vi "SpaceVectorCalc.vi"(0 "ref_alpha":sgl caption="voltage alpha", 1 "Resources":T1={"Multiplier"=refnum, "Divider"=refnum, "Adder"=refnum}, 2 "Parameters":T2={"Deadtime"="Deadtime", "Period"="Period", "A_timing"="A_timing", "B_timing"="B_timing", "C_timing"="C_timing"}, 5 "ref_beta":sgl caption="voltage beta", 7 "ref_max":sgl=1.0) -> (4 "SVPWM_Timing":cluster{"ON":u32, "OFF":u32}[](array[cluster]), 15 "SVPWM_Sector":u8)   [LabVIEW 2017, in "SVPWM.lvlib"]
uses:
  SVPWM.lvlib
  Parameters.ctl
  <vilib>/NI/NonreentrantSinglePoint/Multiplier/Multiplier.lvclass
  <vilib>/NI/NonreentrantSinglePoint/Divider/Divider.lvclass
  <vilib>/NI/NonreentrantSinglePoint/Adder/Adder.lvclass
  <vilib>/rvi/DataTransferAndStorage/Container/Common/niFpgaContainerExecOnDevCompGetState.vi
  <vilib>/rvi/Emulation/niFpgaEmulationIsFPGAContextNoSignature.vi
  <vilib>/rvi/DataTransferAndStorage/Container/Common/niFpgaContainerGetUniqueNameForEmu.vi
  <vilib>/rvi/Memory/Memory_Emulation/niFpgaMemoryEmulationCacheClearOnFirstRun.vi
  <vilib>/rvi/Memory/Memory_Emulation/nirvimemoryEmulationManagerCache_MakeExclusive.vi
  <vilib>/rvi/Memory/Memory_Emulation/niFpgaMemoryEmulationValidateCache.vi
  <vilib>/rvi/Memory/Memory_Emulation/nirvimemoryEmulationManagerCache_InsertValue.vi
  <vilib>/Utility/error.llb/Clear Errors.vi
  <vilib>/rvi/Memory/Memory_Emulation/nirvimemoryEmulationManagerCache_ReleaseExclusive.vi
  <vilib>/rvi/Memory/Memory_Emulation/nirvimemoryEmulationManagerCache_GetValue.vi
  <vilib>/rvi/Memory/Memory_Emulation/nirvimemoryEmulationManagerCache_SetValue.vi
  <vilib>/rvi/Emulation/niFpgaProcessEmulError.vi
  <vilib>/rvi/Emulation/niFpgaSctlEmulationGetInTimedLoop.vi
  <vilib>/rvi/DataTransferAndStorage/Container/XNode/niFpgaContainer.xnode
  <vilib>/rvi/DataTransferAndStorage/Register/Emulation/niFpgaRegisterEmulationRefIn.vi
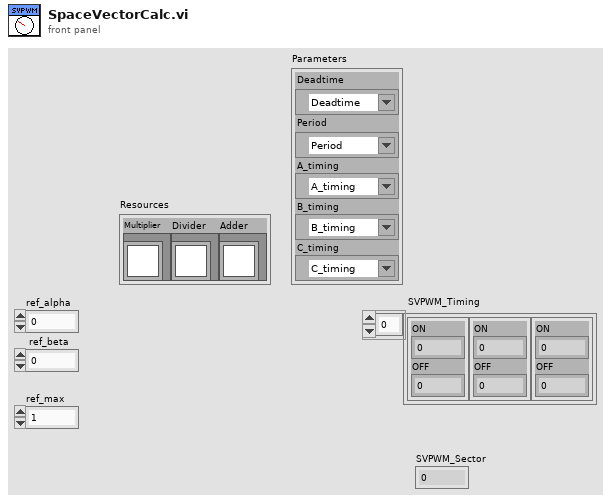
[diagram p1: front panel]
types:
  T1 = cluster{"Multiplier":refnum<class "Multiplier.lvclass">, "Divider":refnum<class "Divider.lvclass">, "Adder":refnum<class "Adder.lvclass">}
  T2 = typedef "SVPWM.lvlib/Parameters.ctl" = cluster{"Deadtime":refnum<k21>, "Period":refnum<k21>, "A_timing":refnum<k21>, "B_timing":refnum<k21>, "C_timing":refnum<k21>}
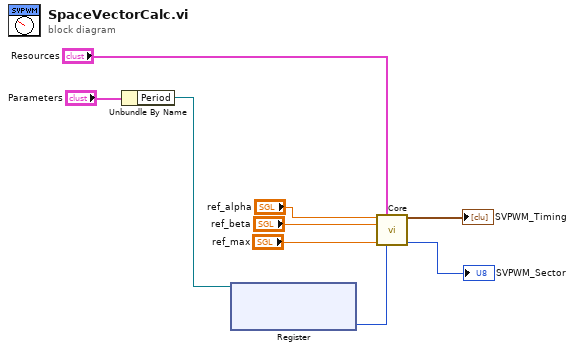
[diagram p0: block diagram]
diagram:
  n1 = Unbundle By Name("Parameters") -> ("Period"=w2:refnum<k21>)
  n2 = xnode "Register"("Register In"=w2) -> ("Data"=w1:u32)  [unwired: 1 out]
  n3 = call "Core.vi"("ref_alpha"="ref_alpha", "Resource"="Resources", "ref_beta"="ref_beta", "ref_max"="ref_max", "Period"=w1) -> ("SVPWM_Timing"=→"SVPWM_Timing":cluster{"ON":u32, "OFF":u32}[], "SVPWM_Sector"=→"SVPWM_Sector":u8)  [unwired: 9 in]
